vi "Day 15-2.vi"() -> ()   [LabVIEW 2019, in "Day 15.lvlib"]
uses:
  Day 15.lvlib
  Controls/Coordenate.ctl
panel:
  out "Min Distance Last Point":u32
  out "Min Distance Matrix":u32[][](array[numeric])
  out "Array":u8[][](array[numeric])
  in  "String":string="1163751742\n1381373672\n2136511328\n3694931569\n7463417111\n1319128137\n1359912421\n3125421639\n1293138521\n2311944581"
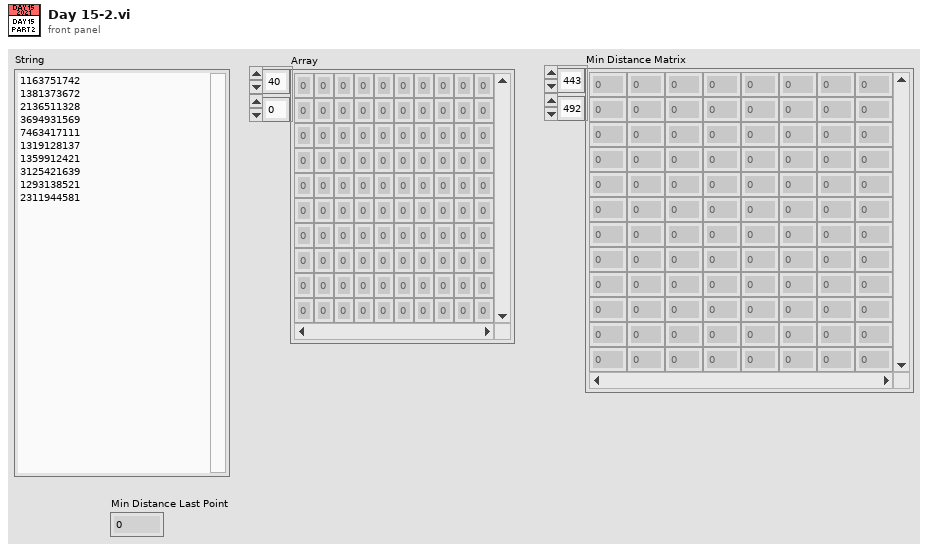
[diagram p1: front panel]
types:
  T1 = typedef "Day 15.lvlib/Coordenate.ctl" = cluster{"Row":i32, "Column":i32}
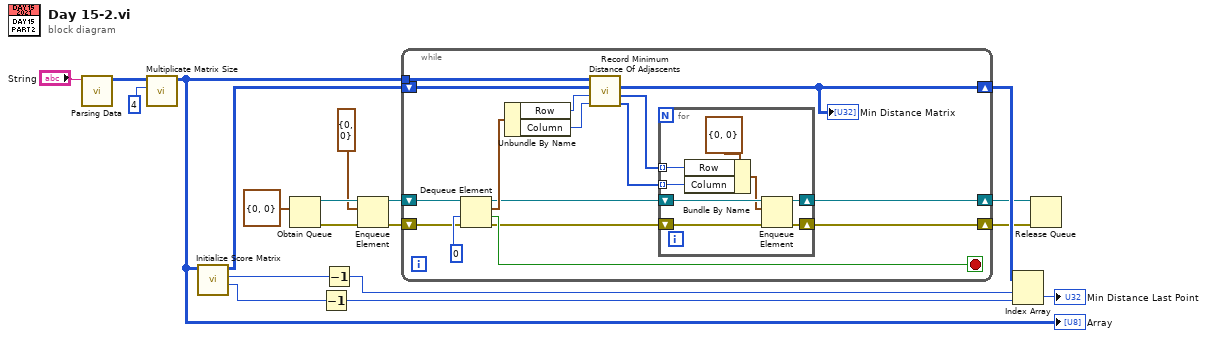
[diagram p0: block diagram]
diagram:
  n1 = call "Parsing Data.vi"("String"="String") -> ("Array"=w3:u8[][])  [unwired: 10 in]
  n2 = call "Multiplicate Matrix Size.vi"("Times to multiply size"=4, "Data Matrix In"=w3) -> ("Data Matrix Out"=w2:u8[][])  [unwired: 9 in]
  "Array" <- w2
  n3 = call "Initialize Score Matrix.vi"("Data Matrix"=w2) -> ("Columns"=w17:i32, "Rows"=w18:i32, "Score Matrix"=w14:u32[][])  [unwired: 8 in]
  n4 = Obtain Queue(element data type=T1 {"Row"=0, "Column"=0} ("Coordenate")) -> (queue out=w10:refnum<queue>, error out=w8:errorcluster)  [unwired: 4 in, 1 out]
  n5 = Decrement(x=w17) -> (x-1=w15:i32)
  n6 = Decrement(x=w18) -> (x-1=w16:i32)
  n7 = Enqueue Element(queue=w10, element=T1 {"Row"=0, "Column"=0}, error in (no error)=w8) -> (queue out=w7:refnum<queue>, error out=w6:errorcluster)  [unwired: 1 in, 1 out]
  n8 = while {
    tunnel: w2 -> [w35]
    shift-right: [w33] -> w13
    shift-left: w14 -> [w34]
    shift-right: [w21] -> w5
    shift-left: w7 -> [w32]
    shift-right: [w20] -> w4
    shift-left: w6 -> [w29]
    stop <- w31 stop-if-true
    n9 = Dequeue Element(queue=w32, timeout in ms (-1)=0, error in (no error)=w29) -> (queue out=w23:refnum<queue>, element=w28:T1, timed out?=w31:bool, error out=w22:errorcluster)
    n10 = Unbundle By Name(w28) -> ("Row"=w27:i32, "Column"=w26:i32)
    n11 = call "Record Minimum Distance Of Adjascents.vi"("Column In"=w26, "Row In"=w27, "Minimum Distance Matrix In"=w34, "Data Matrix"=w35) -> ("Columns Out"=w24:i32[], "Rows Out"=w25:i32[], "Minimum Distance Matrix Out"=w33:u32[][])  [unwired: 5 in]
    "Min Distance Matrix" <- w33
    n12 = for {
      tunnel: w25 -> [w42] mode=indexing
      tunnel: w24 -> [w41] mode=indexing
      shift-right: [w38] -> w21
      shift-left: w23 -> [w39]
      shift-right: [w37] -> w20
      shift-left: w22 -> [w40]
      n13 = Bundle By Name(cluster=T1 {"Row"=0, "Column"=0} ("Coordenate"), "Row"=w42, "Column"=w41) -> (w36:T1)
      n14 = Enqueue Element(queue=w39, element=w36, error in (no error)=w40) -> (queue out=w38:refnum<queue>, error out=w37:errorcluster)  [unwired: 1 in, 1 out]
    }
  }
  n15 = Index Array(array=w13, index (row)=w16, index (col)=w15) -> (element=→"Min Distance Last Point":u32)
  n16 = Release Queue(queue=w5, error in (no error)=w4) -> ()  [unwired: 1 in, 3 out]
